vi "Update Tool Status Helper.vi"(7 "STATUS Cluster in":T1, 8 "error in (no error)":errorcluster, 9 "Trig State in":bool, 10 "OK to Connect":bool, 11 "Connecting":bool) -> (0 "error out":errorcluster, 1 "Trig State out":bool, 2 "Stream Connected":bool, 3 "Status Bits":u32, 5 "STATUS Cluster out":T1)   [LabVIEW 2015, in "Tool Module.lvlib"]
uses:
  Tool Module.lvlib
  _STATUS Typedef--cluster.ctl
  Tool Interface/Tool Interface.lvlib
  <resource>/objmgr/ni.dex.rc
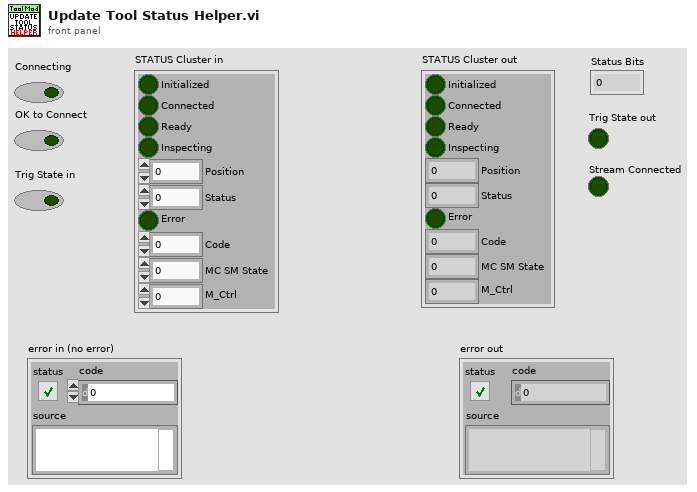
[diagram p1: front panel]
types:
  T1 = typedef "Tool Module.lvlib/_STATUS Typedef--cluster.ctl" = cluster{"Initialized":bool, "Connected":bool, "Ready":bool, "Inspecting":bool, "Position":dbl, "Status":u16, "Error":bool, "Code":i32, "MC SM State":u16, "M_Ctrl":u16}
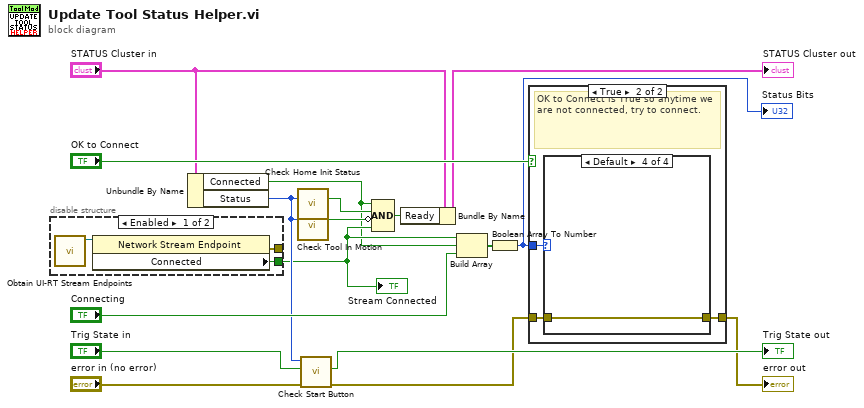
[diagram p0: block diagram]
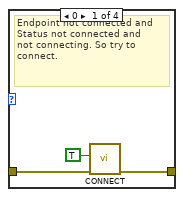
[diagram p3: hidden frame]
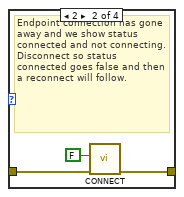
[diagram p4: hidden frame]
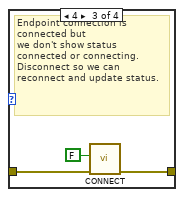
[diagram p5: hidden frame]
diagram:
  n1 = disable-structure shown="Enabled" {
    disable-tunnel: [w19 _] -> w3
    disable-tunnel: [w18 _] -> _
    frame Enabled {
      n2 = call "Obtain UI-RT Stream Endpoints.vi"() -> ("RT Message Stream"=w20:refnum<k21>)  [unwired: 9 in, 2 out]
      n3 = property on="Property Node" class="Network Stream Endpoint"(reference=w20) -> (error out=w18:errorcluster, "Connected"=w19:bool)  [unwired: 1 in, 1 out]
    }
    frame Disabled {
    }
  }
  "Stream Connected" <- w3
  n4 = Unbundle By Name("STATUS Cluster in") -> ("Connected"=w2:bool, "Status"=w8:u16)
  n5 = call "Check Home Init Status.vi"("Status Byte"=w8) -> ("Home Init?"=w14:bool)  [unwired: 14 in]
  n6 = call "Check Tool In Motion.vi"("Status Byte"=w8) -> ("Tool In Motion?"=w15:bool)  [unwired: 14 in]
  n7 = call "Check Start Button.vi"("error in"="error in (no error)", "Trigger Status"="Trig State in", "Status Byte"=w8) -> ("error out"=w5:errorcluster, "Trigger Pressed?"=→"Trig State out":bool)  [unwired: 7 in]
  n8 = Compound Arithmetic op=AND(w2, w14, invert w15, w3) -> (w11:bool)
  n9 = Bundle By Name(cluster="STATUS Cluster in", "Ready"=w11) -> (→"STATUS Cluster out":T1)
  n10 = Build Array(w3, w2, "Connecting") -> (w13:bool[])
  n11 = Boolean Array To Number(Boolean array=w13) -> (number=w1:u32)
  "Status Bits" <- w1
  n12 = case shown="True" "OK to Connect" {
    tunnel: w1 -> [_ w24]
    tunnel: w5 -> [w21 w23]
    tunnel: [w21 w22] -> w9
    frame False {
      # "'OK to Connect' is false, so do nothing."
    }
    frame True {
      # "OK to Connect is True so anytime we are not connected, try to connect."
      n13 = case shown="Default" w24 {
        tunnel: w23 -> [w27 w30 w33 w34]
        tunnel: [w25 w29 w32 w34] -> w22
        frame 0 {
          # "Endpoint not connected and\nStatus not connected and\nnot connecting. So try to connect."
          n14 = call "CONNECT.vi"("error in (no error)"=w27, "Connect"=TRUE) -> ("error out"=w25:errorcluster)  [unwired: 9 in]
        }
        frame 2 {
          # "Endpoint connection has gone away and we show status connected and not connecting.\nDisconnect so status connected goes false and then a reconnect will follow."
          n15 = call "CONNECT.vi"("error in (no error)"=w30, "Connect"=FALSE) -> ("error out"=w29:errorcluster)  [unwired: 9 in]
        }
        frame 4 {
          # "Endpoint connection is connected but\nwe don't show status connected or connecting.\nDisconnect so we can reconnect and update status."
          n16 = call "CONNECT.vi"("error in (no error)"=w33, "Connect"=FALSE) -> ("error out"=w32:errorcluster)  [unwired: 9 in]
        }
        frame Default {
        }
      }
    }
  }
  "error out" <- w9
